vi "json Parse Boolean Array - array path.vi"(8 "error in (no error)":errorcluster, 9 "default":bool[](array[boolean]), 10 "path":string[](array[string]), 11 "JSON Document in":refnum<class "JSON Document.lvclass">) -> (0 "error out":errorcluster, 1 "defaulted?":bool, 2 "value":bool[](array[boolean]), 3 "JSON Document out":refnum<class "JSON Document.lvclass">, 4 "defaulted indices":i32[](array[numeric]))   [LabVIEW 2015, in "JSON Document.lvclass"]
uses:
  JSON Document.lvclass
  json Parse Boolean Array - string path.vi
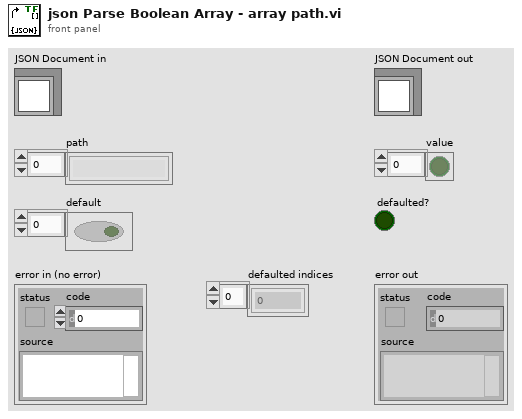
[diagram p1: front panel]
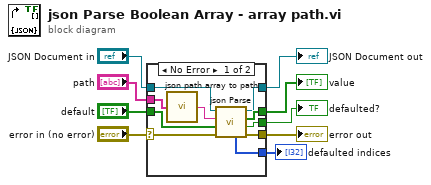
[diagram p0: block diagram]
diagram:
  n1 = case shown="No Error" "error in (no error)" {
    selector: "error in (no error)" -> [w16 w22]
    tunnel: [w15 w22] -> w8
    tunnel: [w12 w21] -> w6
    tunnel: "JSON Document in" -> [w17 w21]
    tunnel: "default" -> [w18 w20]
    tunnel: "path" -> [w19 _]
    tunnel: [w14 w20] -> w3
    tunnel: [w13 _] -> w2
    tunnel: [w10 _] -> w1
    frame No Error {
      n2 = call "json path array to path.vi"("path"=w19) -> ("String"=w11:string)
      n3 = call-poly "json Parse.vi"("error in (no error)"=w16, "default"=w18, "path"=w11, "JSON Document in"=w17) -> ("error out"=w15:errorcluster, "defaulted?"=w13:bool, "value"=w14:bool[], "JSON Document out"=w12:refnum<class "JSON Document.lvclass">, "defaulted indices"=w10:i32[])  [unwired: 3 in]
    }
    frame Error {
    }
  }
  "error out" <- w8
  "JSON Document out" <- w6
  "value" <- w3
  "defaulted?" <- w2
  "defaulted indices" <- w1
